vi "filterPoints.vi"(3 "input":cluster{"x":dbl[], "y":dbl[]}) -> (1 "output":cluster{"x":dbl[], "y":dbl[]})   [LabVIEW 2016]
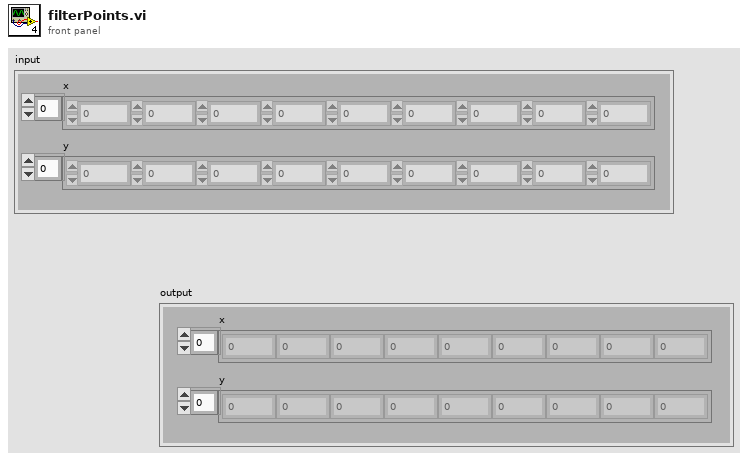
[diagram p1: front panel]
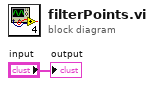
[diagram p0: block diagram]
diagram:
  "output" <- "input"
